vi "movearea.vi"(8 "error in (no error)":errorcluster, 11 "Input":string="y-") -> (0 "error out":errorcluster={"status"=TRUE, "code"=56, "source"="LabVIEWSMTPClient.lvlib:Send.vi:2280002<APPEND>\n\n<b>Complete call chain:</b>\r\n     LabVIEWSMTPClient.lvlib:Send.vi:2280002\r\n     Send Email using SMTP Client.vi:2070001\r\n     movearea.vi\r\n     parse and execute command.vi\r\n     TCPIP.Server v2.vi"}, 3 "Output":string="Approach area changed with 0 crashes ")   [LabVIEW 2014]
uses:
  <userlib>/Nanonis Prog Interface V5/Nanonis Prog Interface.lvlib
  <userlib>/SSL Library/SSL Lib.lvlib
panel:
  in  "Amplitude (V) (Approach":sgl=250.0
  in  "Frequency (Hz) (NaN=no change)":sgl=1000.0
  in  "Amplitude (V) retract":sgl=200.0
  out "num steps z":dbl=500.0
  out "testing?":bool
  out "status":string="approaching"
  in  "STMStatus":T1 {"Size (m)"."Height" format="%.2p"; "Size (m)"."Width" format="%.2p"; "Current (A)" format="%#_6p"; "Z position (m)" format="%#_6p"; "Center coordinates (m)"."Yc" format="%.2p"; "Center coordinates (m)"."Xc" format="%.2p"}
  out "size(s)":i32=1
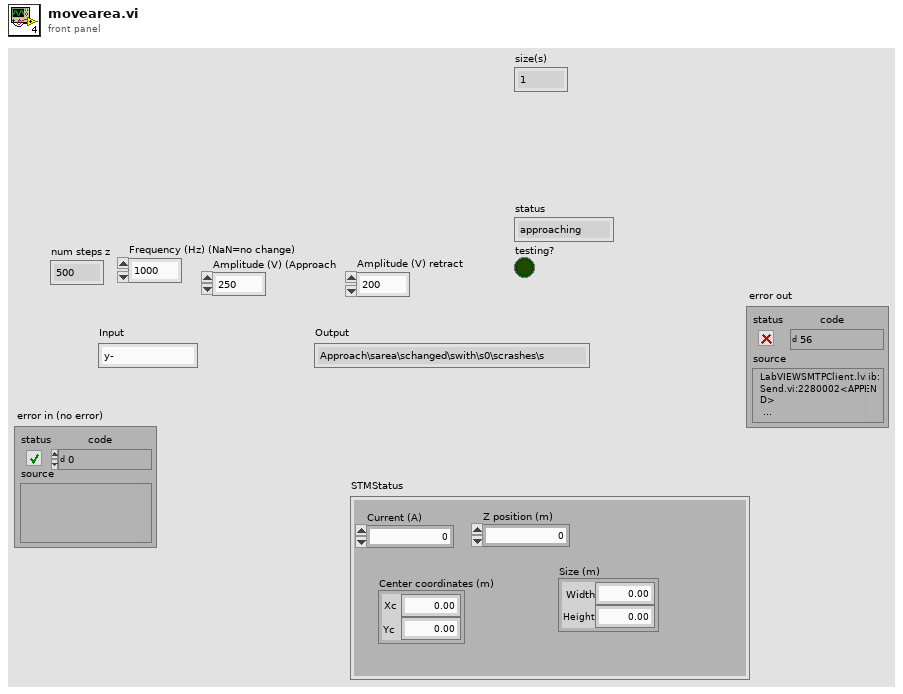
[diagram p1: front panel]
types:
  T1 = cluster{"Center coordinates (m)":cluster{"Xc":sgl, "Yc":sgl}, "Z position (m)":sgl, "Current (A)":sgl, "Size (m)":cluster{"Width":sgl, "Height":sgl}}
  T2 = enum8{"Group 1", "Group 2", "Group 3", "Group 4", "Group 5", "Group 6"}
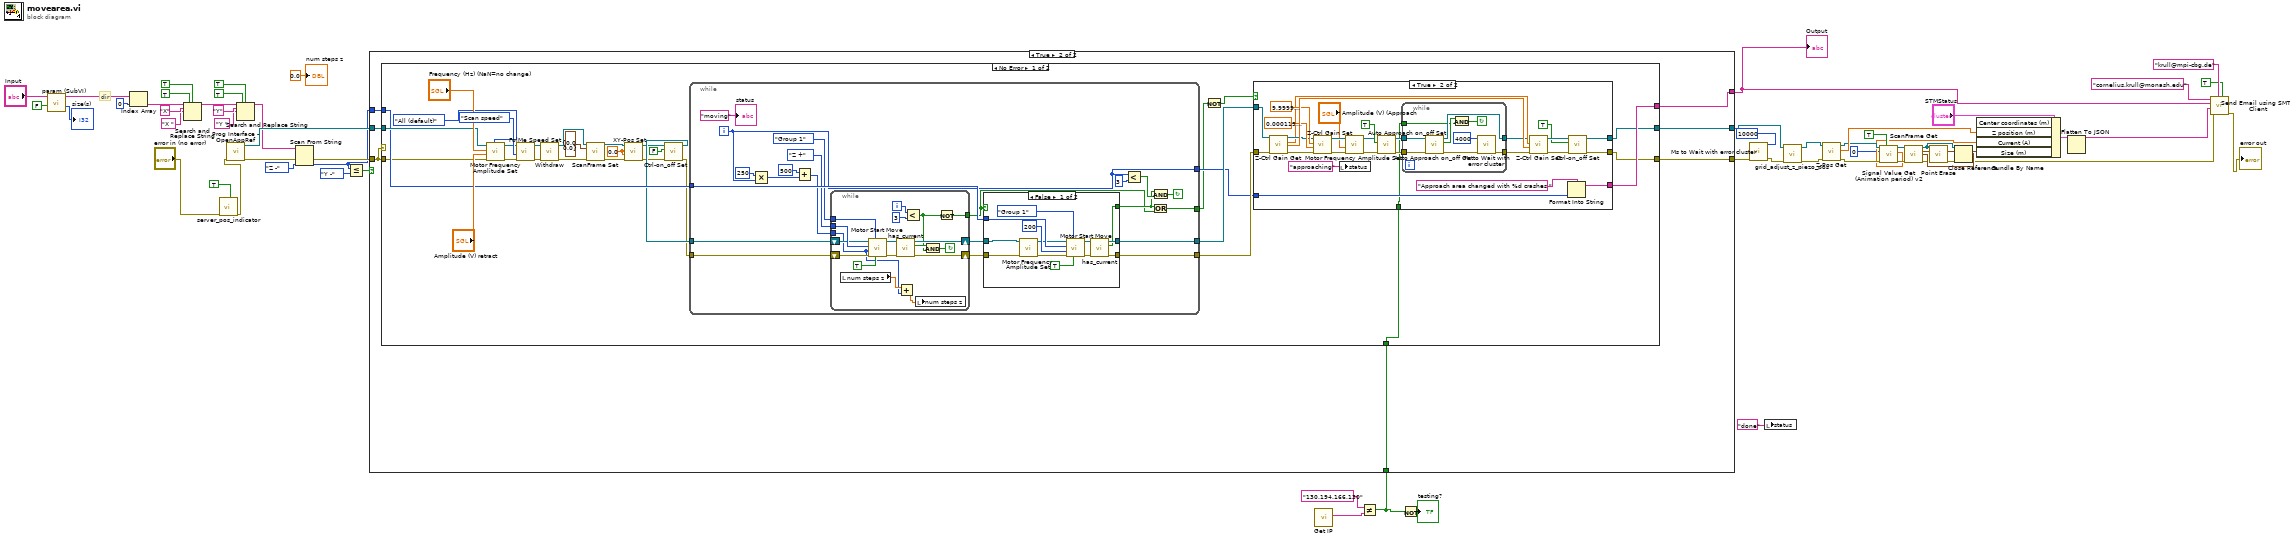
[diagram p0: block diagram]
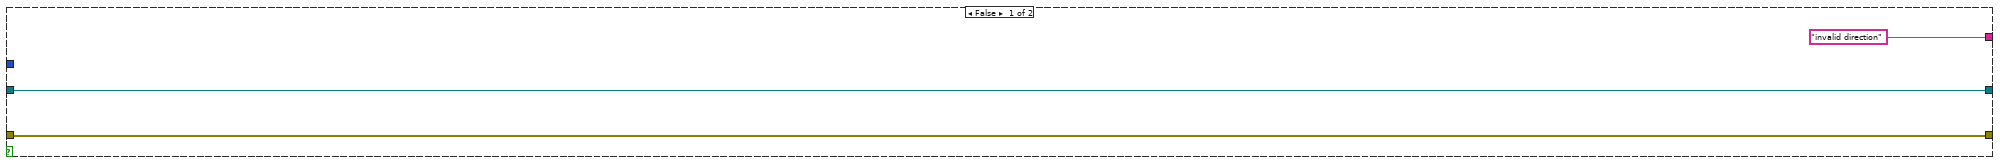
[diagram p2: hidden frame]
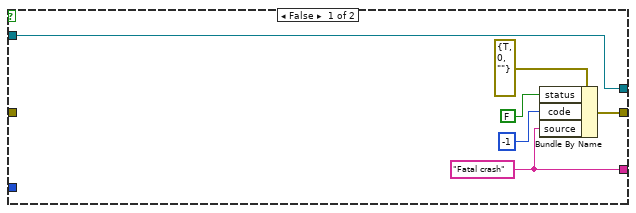
[diagram p3: hidden frame]
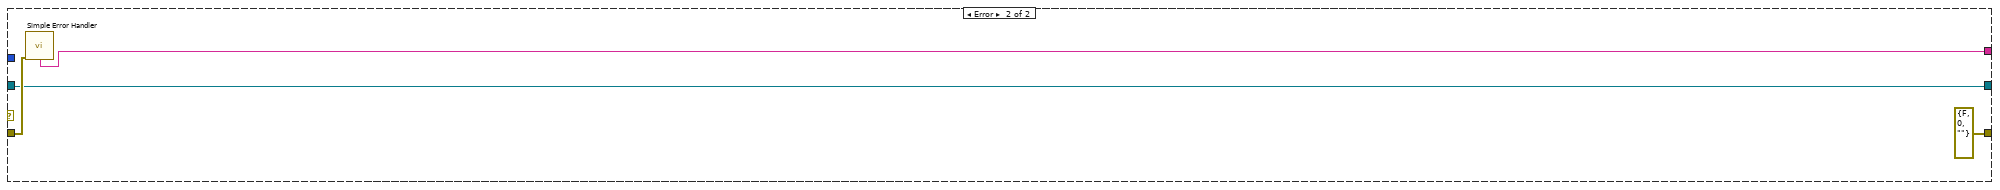
[diagram p5: hidden frame]
diagram:
  # "dir"
  n1 = call <userlib>:"param (SubVI).vi"("Numeric"=FALSE, "Input"="Input") -> ("num"=→"size(s)":i32, "Array"=w57:string[])  [unwired: 7 in, 1 out]
  n2 = Index Array(array=w57, index=0) -> (element=w48:string)
  n3 = Search and Replace String(replace all?=TRUE ("replace all? (F)"), case sensitive?=TRUE ("ignore case? (F)"), input string=w48, search string="X", replace string="X " ("replace string (\"\")")) -> (result string=w39:string)  [unwired: 3 in, 3 out]
  n4 = call "server_pos_indicator.vi"("reset"=TRUE, "error in"="error in (no error)") -> ("error out"=w3:errorcluster)  [unwired: 9 in]
  n5 = call <userlib>:"Prog Interface - OpenAppRef.vi"("Error in (no error)"=w3) -> ("Error out"=w54:errorcluster, "Application reference"=w58:refnum<vi>)  [unwired: 5 in]
  n6 = Search and Replace String(replace all?=TRUE ("replace all? (F)"), case sensitive?=TRUE ("ignore case? (F)"), input string=w39, search string="Y", replace string="Y " ("replace string (\"\")")) -> (result string=w38:string)  [unwired: 3 in, 3 out]
  n7 = Scan From String(input string=w38, error in=w54, default 1=enum16{"X +", "X -", "Y +", "Y -", "Z +", "Z -"}."Z -" ("Direction")) -> (error out=w53:errorcluster, output 1=w52:enum16{"X +", "X -", "Y +", "Y -", "Z +", "Z -"})  [unwired: 2 in, 2 out]
  n8 = Less Or Equal?(x=w52, y=enum16{"X +", "X -", "Y +", "Y -", "Z +", "Z -"}."Y -") -> (x <= y?=w50:bool)
  n9 = call <userlib>:"Get IP.vi"() -> ("IP Address"=w22:string)  [unwired: 10 in, 1 out]
  n10 = Not Equal?(x="130.194.166.130" ("IP Address"), y=w22) -> (x != y?=w20:bool)
  n11 = case shown="True" w50 {
    tunnel: w58 -> [w61 w70]
    tunnel: w52 -> [_ w69]
    tunnel: w53 -> [w63 w68]
    tunnel: [w63 w67] -> w8
    tunnel: ["invalid direction" ("message") w66] -> w17
    tunnel: [w61 w65] -> w7
    tunnel: w20 -> [_ w64]
    frame False {
    }
    frame True {
      n12 = case shown="No Error" w68 {
        tunnel: w70 -> [w89 w200]
        tunnel: w69 -> [w87 _]
        tunnel: w68 -> [w86 w203]
        tunnel: [w73 errorcluster {"status"=FALSE, "code"=0, "source"=""} ("error out")] -> w67
        tunnel: [w78 w202] -> w66
        tunnel: [w72 w200] -> w65
        tunnel: w64 -> [w71 _]
        frame No Error {
          w96 = sgl 0.0 ("X (m)")
          n13 = call <userlib>:"Motor Frequency Amplitude Set.vi"("Axis (All)"=enum16{"All (default)", "X", "Y", "Z"}."All (default)", "Error in (no error)"=w86, "Amplitude (V) (NaN=no change)"="Amplitude (V) retract", "Frequency (Hz) (NaN=no change)"="Frequency (Hz) (NaN=no change)", "Application ref in"=w89) -> ("Error out"=w85:errorcluster, "Application ref out"=w88:refnum<vi>)  [unwired: 5 in]
          n14 = call <userlib>:"FolMe Speed Set.vi"("error in (no error)"=w85, "Speed Setting (Custom)"=enum32{"Scan speed", "Custom speed"}."Scan speed", "Application ref in"=w88) -> ("error out"=w93:errorcluster, "Application ref out"=w94:refnum<vi>)  [unwired: 5 in]
          n15 = call <userlib>:"Withdraw.vi"("Error in (no error)"=w93, "Application ref in"=w94) -> ("Error out"=w100:errorcluster, "Application ref out"=w101:refnum<vi>)  [unwired: 8 in]
          n16 = call <userlib>:"ScanFrame Set.vi"("Application ref in"=w101, "Center coordinates (m)"=cluster{"Xc":sgl, "Yc":sgl} {"Xc"=0.0, "Yc"=0.0}, "error in (no error)"=w100) -> ("Application ref out"=w97:refnum<vi>, "error out"=w98:errorcluster)  [unwired: 11 in]
          n17 = call <userlib>:"XY-Pos Set.vi"("error in (no error)"=w98, "Y (m)"=w96, "X (m)"=w96, "Application ref in"=w97) -> ("error out"=w79:errorcluster, "Application ref out"=w80:refnum<vi>)  [unwired: 4 in]
          n18 = call <userlib>:"Ctrl-on_off Set.vi"("error in (no error)"=w79, "Z Controller ON/OFF"=FALSE, "Application ref in"=w80) -> ("error out"=w81:errorcluster, "Application ref out"=w82:refnum<vi>)  [unwired: 7 in]
          n19 = while {
            tunnel: w87 -> [w165]
            tunnel: [w155] -> w84
            tunnel: [w154] -> w83
            tunnel: w82 -> [w153]
            tunnel: w81 -> [w152]
            tunnel: [w151] -> w77
            tunnel: [w146] -> w76
            i -> [w151]
            stop <- w157 continue-if-true
            n20 = Multiply(x=250, y=w151) -> (x*y=w160:i32)
            n21 = Add(x=u16 500 ("Number of steps"), y=w160) -> (x+y=w162:i32)
            n22 = while {
              tunnel: enum16{"X +", "X -", "Y +", "Y -", "Z +", "Z -"}."Z +" ("Direction") -> [w199]
              tunnel: T2."Group 1" ("Group") -> [w197]
              tunnel: w162 -> [w183]
              shift-right: [w194] -> w148
              shift-left: w153 -> [w196]
              shift-right: [w191] -> w147
              shift-left: w152 -> [w195]
              tunnel: [w185] -> w145
              i -> [w189]
              stop <- w187 continue-if-true
              n23 = local read "num steps z"() -> (w184:dbl)
              n24 = call <userlib>:"Motor Start Move.vi"("Wait until finished? (F)"=TRUE, "Group"=w197, "Error in (no error)"=w195, "Number of steps"=w183, "Direction"=w199, "Application ref in"=w196) -> ("Error out"=w192:errorcluster, "Application ref out"=w193:refnum<vi>)  [unwired: 3 in]
              n25 = call "has_current.vi"("error in (no error)"=w192, "Application in"=w193) -> ("error out"=w191:errorcluster, "Boolean"=w188:bool, "Application out"=w194:refnum<vi>)  [unwired: 7 in]
              n26 = Add(x=w184, y=w183) -> (x+y=w182:dbl)
              n27 = Less?(x=w189, y=3) -> (x < y?=w186:bool)
              n28 = local write "num steps z"(w182) -> ()
              n29 = And(x=w188, y=w186) -> (x .and. y?=w187:bool)
              n30 = Not(x=w186) -> (.not. x?=w185:bool)
            }
            n31 = case shown="False" w145 {
              selector: w145 -> [_ w179]
              tunnel: w165 -> [w178 _]
              tunnel: [w172 w180] -> w155
              tunnel: [w171 w181] -> w154
              tunnel: [w170 w179] -> w150
              tunnel: w148 -> [w167 w180]
              tunnel: w147 -> [w166 w181]
              frame False {
                n32 = call <userlib>:"Motor Frequency Amplitude Set.vi"("Error in (no error)"=w166, "Application ref in"=w167) -> ("Error out"=w168:errorcluster, "Application ref out"=w169:refnum<vi>)  [unwired: 8 in]
                n33 = call <userlib>:"Motor Start Move.vi"("Wait until finished? (F)"=TRUE, "Group"=T2."Group 1", "Error in (no error)"=w168, "Number of steps"=u16 200, "Direction"=w178, "Application ref in"=w169) -> ("Error out"=w173:errorcluster, "Application ref out"=w174:refnum<vi>)  [unwired: 3 in]
                n34 = call "has_current.vi"("error in (no error)"=w173, "Application in"=w174) -> ("error out"=w171:errorcluster, "Boolean"=w170:bool, "Application out"=w172:refnum<vi>)  [unwired: 7 in]
              }
              frame True {
              }
            }
            n35 = Less?(x=w151, y=3) -> (x < y?=w156:bool)
            n36 = Or(x=w150, y=w145) -> (x .or. y?=w146:bool)
            n37 = And(x=w150, y=w156) -> (x .and. y?=w157:bool)
            "status" <- "moving"
          }
          n38 = Not(x=w76) -> (.not. x?=w75:bool)
          n39 = case shown="True" w75 {
            tunnel: w84 -> [w102 w135]
            tunnel: w83 -> [_ w126]
            tunnel: [w104 w119] -> w78
            tunnel: w77 -> [_ w118]
            tunnel: [w103 w116] -> w73
            tunnel: [w102 w115] -> w72
            tunnel: w71 -> [_ w113]
            frame False {
              w104 = "Fatal crash"
              n40 = Bundle By Name(cluster=errorcluster {"status"=TRUE, "code"=0, "source"=""} ("error out"), "status"=FALSE, "code"=-1, "source"=w104) -> (w103:errorcluster)
            }
            frame True {
              n41 = call <userlib>:"Z-Ctrl Gain Get.vi"("Application ref in"=w135, "error in (no error)"=w126) -> ("Application ref out"=w131:refnum<vi>, "P-gain"=w130:sgl, "Time constant (s)"=w134:sgl, "error out"=w125:errorcluster)  [unwired: 9 in, 1 out]
              n42 = call <userlib>:"Z-Ctrl Gain Set.vi"("error in (no error)"=w125, "Time constant (s)"=sgl 0.00012, "P-gain"=sgl 1e-11, "Application ref in"=w131) -> ("error out"=w111:errorcluster, "Application ref out"=w112:refnum<vi>)  [unwired: 5 in]
              n43 = local write "status"("approaching" ("status")) -> ()
              n44 = call <userlib>:"Motor Frequency Amplitude Set.vi"("Error in (no error)"=w111, "Amplitude (V) (NaN=no change)"="Amplitude (V) (Approach", "Application ref in"=w112) -> ("Error out"=w109:errorcluster, "Application ref out"=w110:refnum<vi>)  [unwired: 7 in]
              n45 = call <userlib>:"Auto Approach on_off Set.vi"("Error in (no error)"=w109, "Auto approach start/stop (F)"=TRUE, "Application ref in"=w110) -> ("Error out"=w124:errorcluster, "Application ref out"=w128:refnum<vi>)  [unwired: 5 in]
              n46 = while {
                tunnel: w128 -> [w142]
                tunnel: [w141] -> w127
                tunnel: w124 -> [w140]
                tunnel: [w139] -> w123
                tunnel: w113 -> [w136]
                stop <- w137 continue-if-true
                n47 = call <userlib>:"Auto Approach on_off Get.vi"("Error in (no error)"=w140, "Application ref in"=w142) -> ("Error out"=w143:errorcluster, "Auto approach on/off status"=w138:bool, "Application ref out"=w141:refnum<vi>)  [unwired: 5 in]
                n48 = And(x=w138, y=w136) -> (x .and. y?=w137:bool)
                n49 = call <userlib>:"Ms to Wait with error cluster.vi"("error in (no error)"=w143, "milliseconds to wait"=u32 4000) -> ("error out"=w139:errorcluster)  [unwired: 4 in, 1 out]
              }
              n50 = call <userlib>:"Z-Ctrl Gain Set.vi"("error in (no error)"=w123, "Time constant (s)"=w134, "P-gain"=w130, "Application ref in"=w127) -> ("error out"=w120:errorcluster, "Application ref out"=w122:refnum<vi>)  [unwired: 5 in]
              n51 = Format Into String(format string="Approach area changed with %d crashes " ("initial string"), w118) -> (resulting string=w119:string)  [unwired: 2 in, 1 out]
              n52 = call <userlib>:"Ctrl-on_off Set.vi"("error in (no error)"=w120, "Z Controller ON/OFF"=TRUE, "Application ref in"=w122) -> ("error out"=w116:errorcluster, "Application ref out"=w115:refnum<vi>)  [unwired: 7 in]
            }
          }
        }
        frame Error {
          n53 = call <vilib>:"Simple Error Handler.vi"("error in (no error)"=w203) -> ("message"=w202:string)  [unwired: 4 in, 4 out]
        }
      }
    }
  }
  "Output" <- w17
  n54 = Not(x=w20) -> (.not. x?=→"testing?":bool)
  n55 = call <userlib>:"Ms to Wait with error cluster.vi"("error in (no error)"=w8, "milliseconds to wait"=u32 10000) -> ("error out"=w10:errorcluster)  [unwired: 4 in, 1 out]
  n56 = local write "status"("done" ("status")) -> ()
  n57 = call "grid_adjust_z_piezo_pos.vi"("Error in (no error)"=w10, "Application ref in"=w7) -> ("Error out"=w9:errorcluster, "Application ref out"=w6:refnum<vi>)  [unwired: 8 in]
  n58 = call <userlib>:"Z-Pos Get.vi"("error in (no error)"=w9, "Application ref in"=w6) -> ("error out"=w29:errorcluster, "Z position (m)"=w35:sgl, "Application ref out"=w32:refnum<vi>)  [unwired: 7 in]
  n59 = call <userlib>:"Signal Value Get (Animation period) v2.vi"("Wait for newest data (F=False)"=TRUE, "error in (no error)"=w29, "Signal index (0-79)"=i8 0, "Application ref in"=w32) -> ("error out"=w30:errorcluster, "Signal value"=w27:sgl, "Application ref out"=w31:refnum<vi>)  [unwired: 4 in]
  n60 = call <userlib>:"ScanFrame Get.vi"("Application ref in"=w31, "error in (no error)"=w30) -> ("Application ref out"=w12:refnum<vi>, "Center coordinates (m)"=w34:cluster{"Xc":sgl, "Yc":sgl}, "Size (m)"=w33:cluster{"Width":sgl, "Height":sgl}, "error out"=w13:errorcluster)  [unwired: 9 in, 1 out]
  n61 = call <userlib>:"Point Erase.vi"("Application ref in"=w12, "error in (no error)"=w13) -> ("error out"=w14:errorcluster)  [unwired: 12 in, 1 out]
  n62 = Close Reference(reference=w12, error in (no error)=w14) -> (error out=w15:errorcluster)
  n63 = Bundle By Name(cluster="STMStatus", "Center coordinates (m)"=w34, "Z position (m)"=w35, "Current (A)"=w27, "Size (m)"=w33) -> (w36:T1)
  n64 = Flatten To JSON(anything=w36) -> (JSON string=w16:string)  [unwired: 2 in, 1 out]
  n65 = call "Send Email using SMTP Client.vi"("send map"=TRUE, "CC"="krull@mpi-cbg.de", "error in (no error)"=w15, "Message"=w16, "Subject"=w17, "To:"="cornelius.krull@monash.edu" ("Recipients")) -> ("error out"=→"error out":errorcluster)  [unwired: 5 in]
  "num steps z" <- 0.0 ("num steps z")
